vi "Set Window Color.vi"() -> ()   [LabVIEW 2020]
panel:
  in  "布尔":bool
  in  "字符串":string
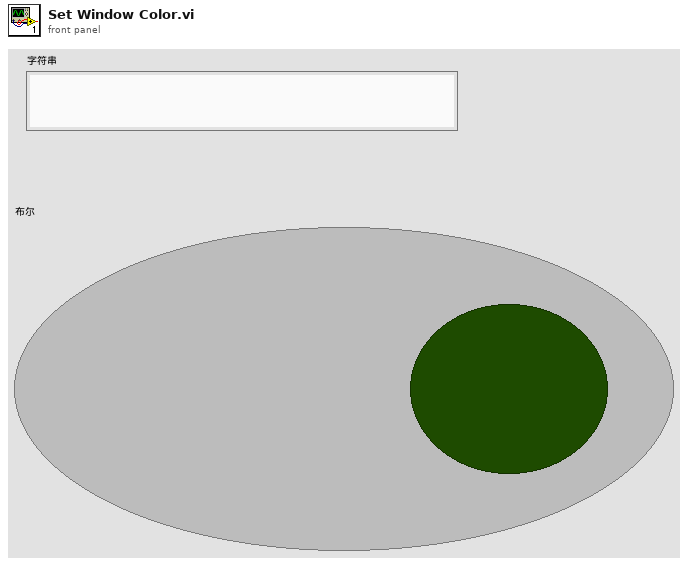
[diagram p1: front panel]
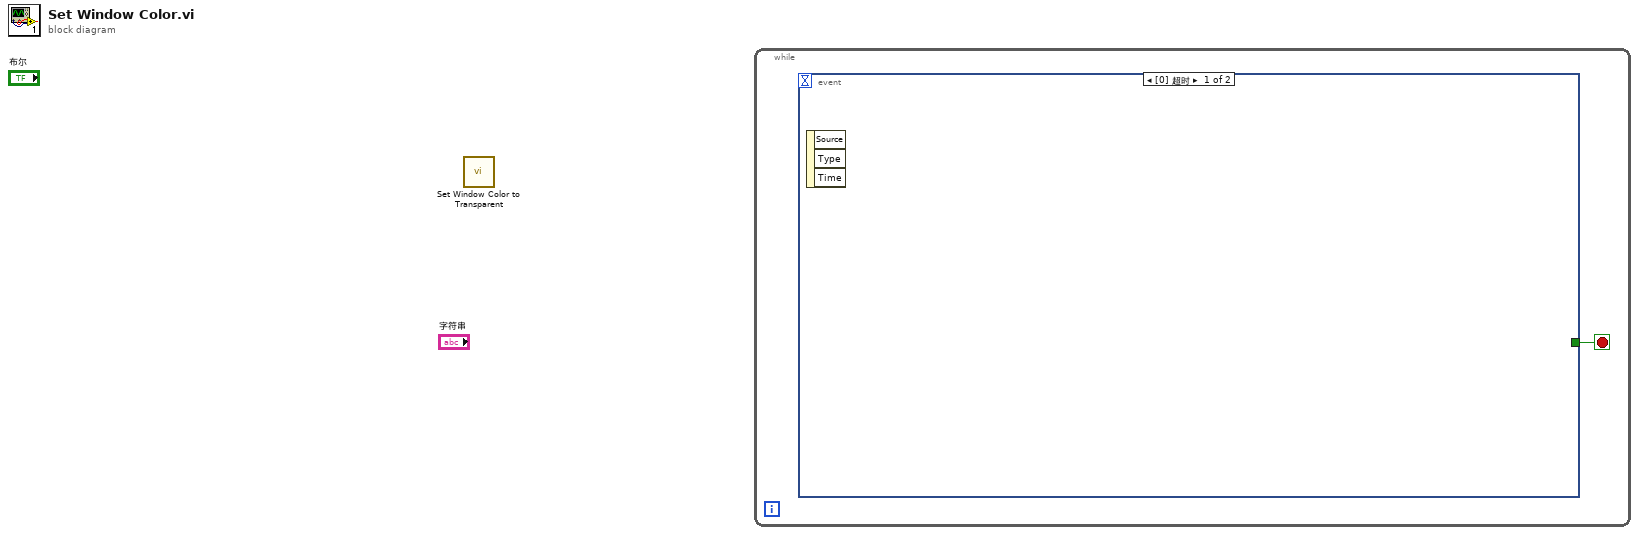
[diagram p0: block diagram]
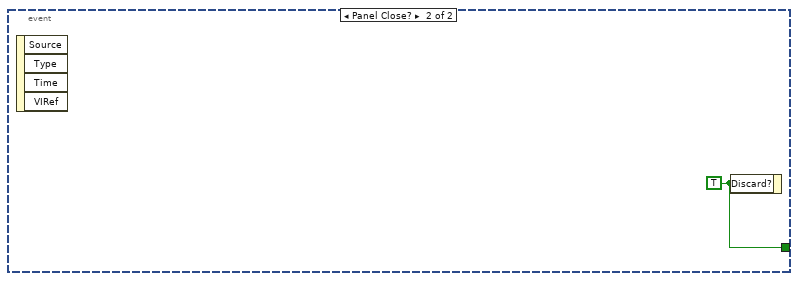
[diagram p2: hidden frame]
diagram:
  n1 = call "Set Window Color to Transparent.vi"() -> ()  [unwired: 8 in, 1 out]
  n2 = while {
    stop <- w1 stop-if-true
    n3 = event shown="[0] 超时" {
      selector: _ -> [_ _]
      dyn-events: _ -> [_ _]
      timeout: _ -> [_ _]
      tunnel: [_ w2] -> w1
      event Timeout {
        n4 = event-data() -> ()  [unwired: 1 in, 3 out]
      }
      event Panel Close? {
        w2 = TRUE ("放弃？")
        n5 = event-data() -> ()  [unwired: 1 in, 4 out]
        n6 = event-data("Discard?"=w2) -> ()  [unwired: 1 in, 1 out]
      }
    }
  }
